vi "Get Timing Information.vi"(8 "Error In":errorcluster, 10 "Binary Data":u8[](array[numeric]), 11 "Number of Pages":i32) -> (0 "Error Out":errorcluster, 1 "Time Axis":dbl[](array[numeric]), 2 "End Time":timestamp, 3 "Start Time":timestamp)   [LabVIEW 2017]
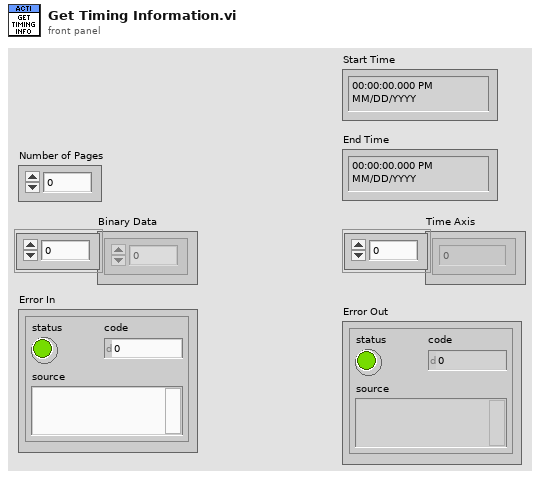
[diagram p1: front panel]
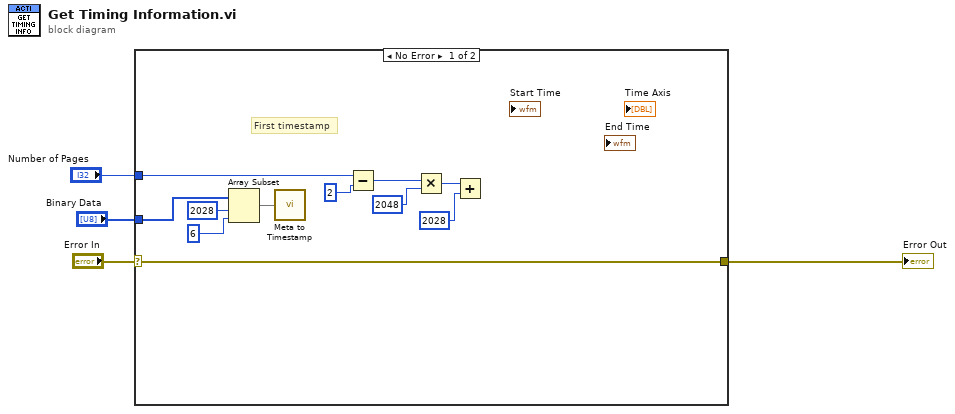
[diagram p0: block diagram]
diagram:
  n1 = case shown="No Error" "Error In" {
    selector: "Error In" -> [w15 _]
    tunnel: [w15 _] -> w3
    tunnel: "Number of Pages" -> [w10 _]
    tunnel: "Binary Data" -> [w12 _]
    frame No Error {
      # "First timestamp"
      n2 = Array Subset(array=w12, index=2028, length=6) -> (w11:u8[])
      n3 = call "Meta to Timestamp.vi"("binaryTimestampWithOffset"=w11) -> ()  [unwired: 2 out]
      n4 = Subtract(x=w10, y=2) -> (x-y=w8:i32)
      n5 = Multiply(x=w8, y=2048) -> (x*y=w6:i32)
      n6 = Add(x=w6, y=2028) -> ()  [unwired: 1 out]
    }
    frame Error {
    }
  }
  "Error Out" <- w3
